vi "GetLogFormatter.vi"(8 "Error in (no error)":errorcluster, 11 "LogWriterInterface in":refnum<class "LogWriterInterface.lvclass">) -> (0 "Error out":errorcluster, 2 "LogFormatterInterface out":refnum<class "LogFormatterInterface.lvclass">, 3 "LogWriterInterface out":refnum<class "LogWriterInterface.lvclass">)   [LabVIEW 2011, in "LogWriterInterface.lvclass"]
uses:
  LogWriterInterface.lvclass
  Formatter/LogFormatterInterface/LogFormatterInterface.lvclass
  LogWriterInterface.lvclass/LogWriterInterface.ctl
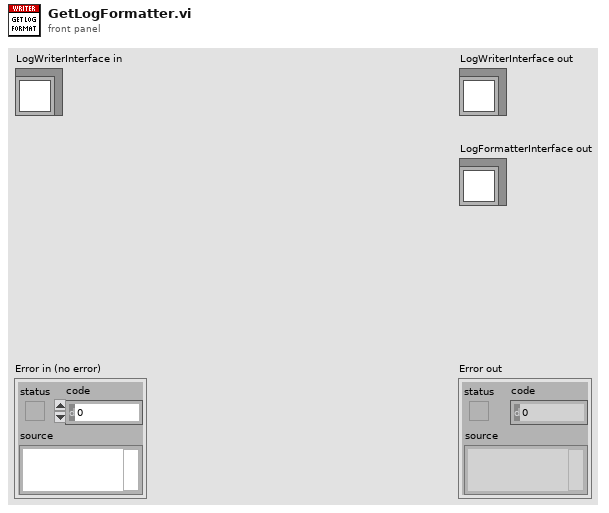
[diagram p1: front panel]
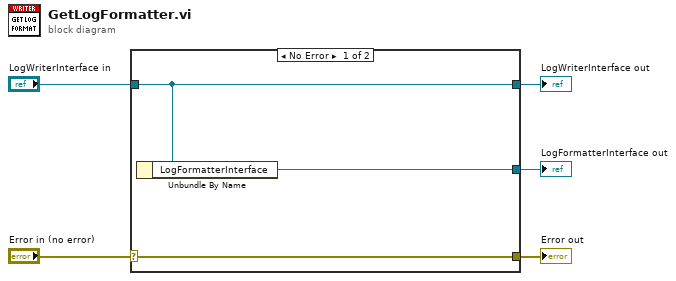
[diagram p0: block diagram]
diagram:
  n1 = case shown="No Error" "Error in (no error)" {
    selector: "Error in (no error)" -> [w8 w9]
    tunnel: [w8 w9] -> w4
    tunnel: [w7 w10] -> w2
    tunnel: "LogWriterInterface in" -> [w7 w10]
    tunnel: [w6 _] -> w1
    frame No Error {
      n2 = Unbundle By Name(w7) -> ("LogFormatterInterface"=w6:refnum<class "LogFormatterInterface.lvclass">)
    }
    frame Error {
    }
  }
  "Error out" <- w4
  "LogWriterInterface out" <- w2
  "LogFormatterInterface out" <- w1
